vi "Util_RoundsToMeters.vi"(10 "rounds gear":dbl) -> (2 "distance (m) robot":dbl)   [LabVIEW 2009, in "OWNCAN.lvlib"]
uses:
  OWNCAN.lvlib
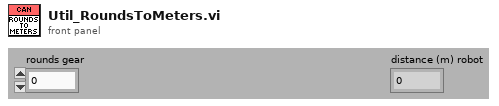
[diagram p1: front panel]
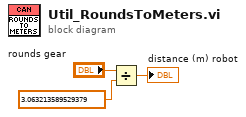
[diagram p0: block diagram]
diagram:
  n1 = Divide(x="rounds gear", y=3.063213589529379) -> (x/y=→"distance (m) robot":dbl)
